vi "Set Zero Position (SubVI).vi"(7 "Device Address In":i32, 8 "entrée d'erreur (pas d'erreur)":errorcluster, 9 "DeviceKey In":string, 10 "Motor":i32, 11 "Refnum de .NET en entrée":refnum<k24>) -> (0 "sortie d'erreur":errorcluster, 1 "DeviceKey Out":string, 2 "Device Address Out":i32, 3 "Refnum de .NET en sortie":refnum<k24>)   [LabVIEW 2017]
doc: "by Tanguy BOULARD"
uses:
  dll/CmdLib.dll
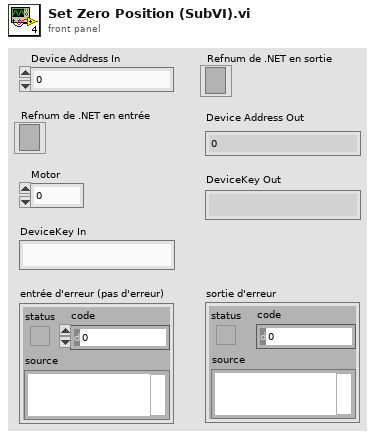
[diagram p1: front panel]
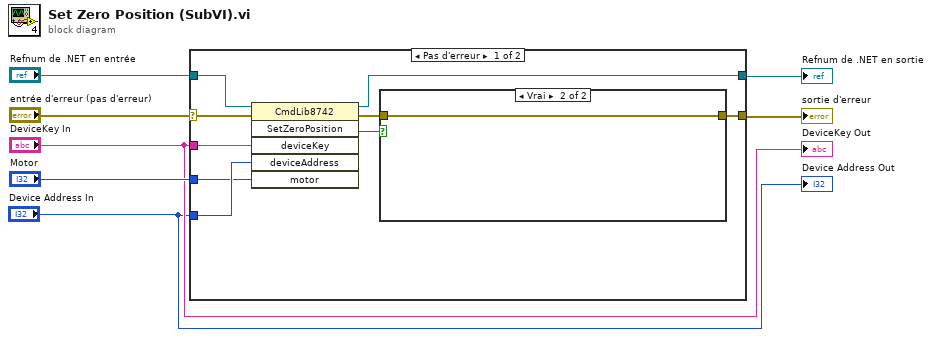
[diagram p0: block diagram]
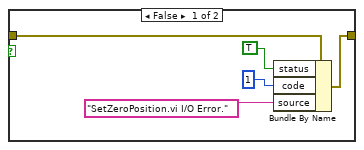
[diagram p2: hidden frame]
diagram:
  n1 = case shown="Pas d'erreur" "entrée d'erreur (pas d'erreur)" {
    selector: "entrée d'erreur (pas d'erreur)" -> [w13 w23]
    tunnel: "Refnum de .NET en entrée" -> [w16 w24]
    tunnel: [w15 w24] -> w4
    tunnel: "Motor" -> [w8 _]
    tunnel: "DeviceKey In" -> [w14 _]
    tunnel: [w10 w23] -> w6
    tunnel: "Device Address In" -> [w9 _]
    frame No Error {
      n2 = invoke class="CmdLib8742" method="SetZeroPosition"(reference=w16, error in=w13, "deviceKey"=w14, "deviceAddress"=w9, "motor"=w8) -> (reference out=w15:refnum<k24>, error out=w11:errorcluster, "SetZeroPosition"=w12:bool)  [unwired: 1 in, 3 out]
      n3 = case shown="Vrai" w12 {
        tunnel: w11 -> [w21 w22]
        tunnel: [w20 w22] -> w10
        frame False {
          n4 = Bundle By Name(cluster=w21, "status"=TRUE, "code"=1, "source"="SetZeroPosition.vi I/O Error.") -> (w20:errorcluster)
        }
        frame True {
        }
      }
    }
    frame Error {
    }
  }
  "sortie d'erreur" <- w6
  "Refnum de .NET en sortie" <- w4
  "DeviceKey Out" <- "DeviceKey In"
  "Device Address Out" <- "Device Address In"
